vi "Close.vi"(8 "error in":errorcluster, 11 "Web App Handle":T1) -> (0 "error out":errorcluster)   [LabVIEW 2013, in "Web Messaging API.lvlib"]
doc: "Closes the Web Messaging connection"
uses:
  Web Messaging API.lvlib
  Web Messaging Handle.ctl
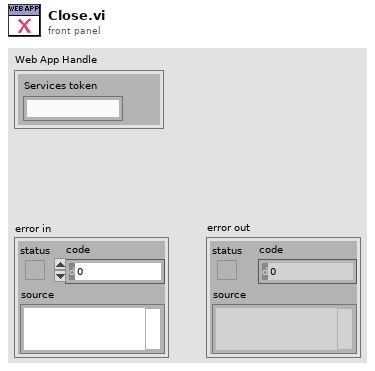
[diagram p1: front panel]
types:
  T1 = typedef "Web Messaging API.lvlib/Web Messaging Handle.ctl" = cluster{"Services token":string}
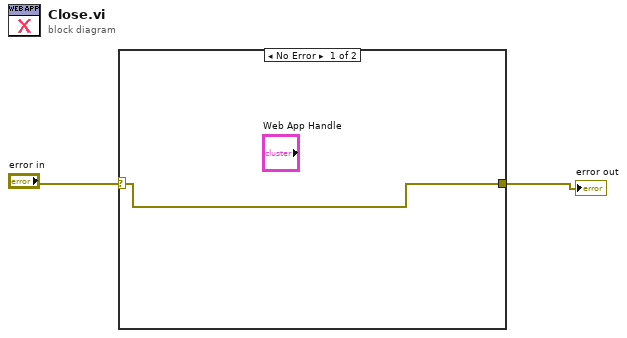
[diagram p0: block diagram]
diagram:
  n1 = case shown="No Error" "error in" {
    selector: "error in" -> [w3 w4]
    tunnel: [w3 w4] -> w2
    frame No Error {
    }
    frame Error {
    }
  }
  "error out" <- w2
